vi "Proc_DCS.vi"(11 "error in (no error)":errorcluster, 12 "log file":path=path "/home/ArcVIEW/Logs/MOD_Logic_DCS.log", 13 "Database RefNum out":T1) -> (15 "error out":errorcluster)   [LabVIEW 2016]
uses:
  DBSHAND/private/vis/DatabaseHand_RefNum.ctl
  Common/public/vis/CMN_FVAR_action.ctl
  DBSHAND/private/vis/DatabaseHand_Element_Get(bool).vi
panel:
  out "queue":T2
  out "occurrence":refnum<k4>
  in  "input ptrs":u64[](array[numeric])
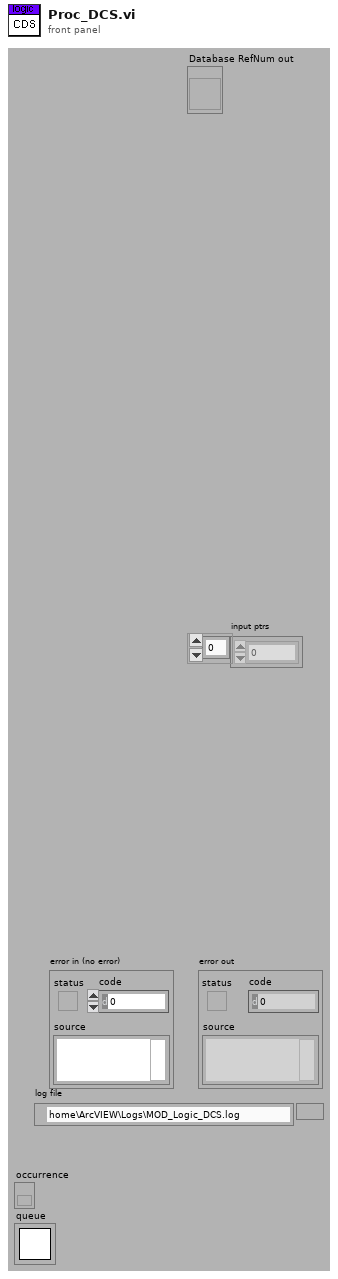
[diagram p1: front panel]
types:
  T1 = typedef "DatabaseHand_RefNum.ctl" = refnum<vi>
  T2 = typedef "Queue RefNum" = refnum<k1>
  T3 = typedef "CMN_FVAR_action.ctl" = enum16{"read", "write"}
  T4 = typedef "CMN_ContStatus.ctl" = cluster{"Response":string, "power":bool, "shutter":bool, "artifdata":bool, "idlemode":bool, "reset":bool, "gain":u8, "speed":u8, "resetPCI":bool, "autoshutter":bool, "TempSetPoint":i32, "multipleextensions":bool, "displayImage":bool, "coadding":bool, "images being coadded":i32, "Operation Mode":enum16{"normal", "coadd", "fawler"}, "frames to write":cluster{"subs":bool, "reset":bool, "exposed":bool}, "fawler samples":i32, "write auto":bool, "datatype":string, "frames to display":cluster{"subs":bool, "reset":bool, "exposed":bool}, "sur":i32, "autoclear":bool}
  T5 = typedef "CMN_Buffers.ctl" = cluster{"TotalPixels":u32, "Total image bytes":u32, "Total Phys Buffers":u32, "virtual buf pixels":u32, "virtual bytes size":u32, "Remaining piece":u32, "Transfer_Buf_size":u32}
  T6 = cluster{"subs":bool, "reset":bool, "exposed":bool}
  T7 = cluster{"name":string, "number":i32, "bpp":u8, "write ":bool, "imageToRead":u16, "rootName":string}
  T8 = cluster{"pointer":u64, "size":u64, "progress":u32, "status":string}
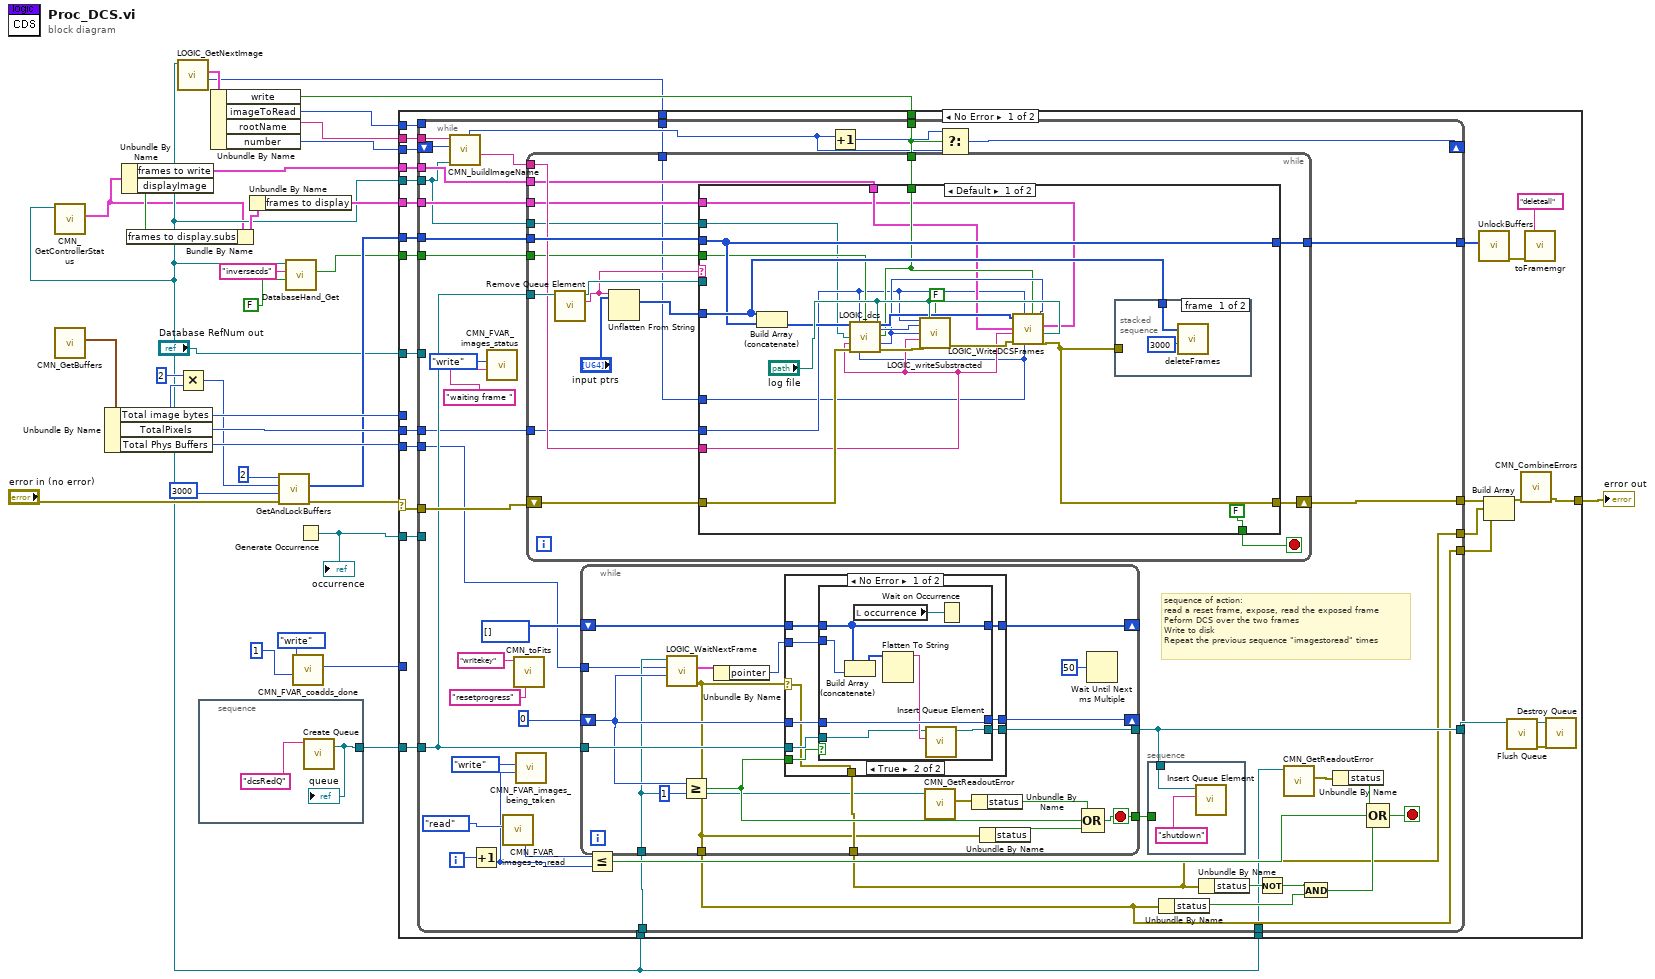
[diagram p0: block diagram]
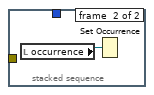
[diagram p2: hidden frame]
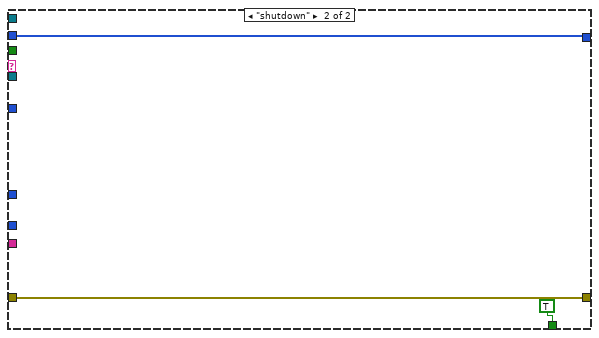
[diagram p3: hidden frame]
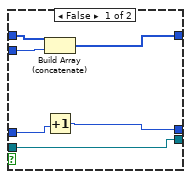
[diagram p4: hidden frame]
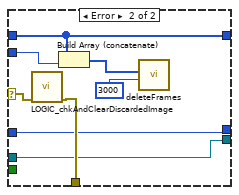
[diagram p5: hidden frame]
diagram:
  n1 = call "CMN_GetControllerStatus.vi"("DBS Ref"="Database RefNum out") -> ("ControllerStatus"=w3:T4)  [unwired: 10 out]
  n2 = call "CMN_GetBuffers.vi"() -> ("BuffersDimensions"=w5:T5)  [unwired: 2 in, 9 out]
  n3 = Unbundle By Name(w5) -> ("Total image bytes"=w28:u32, "TotalPixels"=w31:u32, "Total Phys Buffers"=w29:u32)
  n4 = Unbundle By Name(w3) -> ("frames to write"=w32:T6, "displayImage"=w14:bool)
  n5 = Bundle By Name(cluster=w3, "frames to display.subs"=w14) -> (w13:T4)
  n6 = call "LOGIC_GetNextImage.vi"("DBS Ref"="Database RefNum out") -> ("raw bpp"=w2:i32, "next image info"=w6:T7)  [unwired: 9 out]
  n7 = Multiply(x=u32 2, y=w28) -> (x*y=w24:u32)
  n8 = stacked-sequence {
    tunnel: [w33] -> w19
    frame #0 {
      n9 = call <vilib>:"Create Queue.vi"("name (unnamed)"="dcsRedQ") -> ("queue out"=w33:T2)  [unwired: 3 in, 3 out]
      "queue" <- w33
    }
  }
  n10 = Unbundle By Name(w6) -> ("write"=w17:bool, "imageToRead"=w18:u16, "rootName"=w16:string, "number"=w15:i32)
  n11 = Unbundle By Name(w13) -> ("frames to display"=w12:T6)
  n12 = call "GetAndLockBuffers.vi"("error in"="error in (no error)", "ms timeout (-1)"=3000, "size"=w24, "amount of buffers"=u16 2) -> ("error out"=w20:errorcluster, "ptrs"=w22:u64[])  [unwired: 1 in, 5 out]
  n13 = call-poly "DatabaseHand_Get.vi"("default value"=FALSE, "name"="inversecds", "Database RefNum in"="Database RefNum out") -> ("value"=w9:bool)  [unwired: 2 in, 6 out]
  n14 = call "CMN_FVAR_coadds_done.vi"("value in"=u16 1 ("images coadded"), "action"=CMN_FVAR_action."write") -> ("value out"=w1:i32)  [unwired: 8 out]
  n15 = Generate Occurrence() -> (w26:refnum<k4>)
  "occurrence" <- w26
  n16 = case shown="No Error" w20 {
    selector: w20 -> [w63 w205]
    tunnel: w32 -> [w58 _]
    tunnel: w31 -> [w36 _]
    tunnel: [w47 w205] -> w30
    tunnel: w29 -> [w53 _]
    tunnel: w26 -> [w59 _]
    tunnel: w22 -> [w62 _]
    tunnel: w19 -> [w60 _]
    tunnel: w28 -> [_ _]
    tunnel: w18 -> [w57 _]
    tunnel: w17 -> [w46 _]
    tunnel: "Database RefNum out" -> [w44 _]
    tunnel: "Database RefNum out" -> [w43 _]
    tunnel: "Database RefNum out" -> [w42 _]
    tunnel: w16 -> [w41 _]
    tunnel: w15 -> [w40 _]
    tunnel: w12 -> [w39 _]
    tunnel: w9 -> [w38 _]
    tunnel: "Database RefNum out" -> [w37 _]
    tunnel: w2 -> [w35 _]
    tunnel: w1 -> [_ _]
    frame No Error {
      n17 = while {
        tunnel: [w88] -> w45
        tunnel: w46 -> [w87]
        tunnel: [w91] -> w49
        tunnel: w53 -> [w65]
        tunnel: w57 -> [_]
        tunnel: w58 -> [w75]
        tunnel: w59 -> [_]
        tunnel: [w95] -> w56
        tunnel: w60 -> [w96]
        shift-left: w40 -> [w78]
        shift-right: [w85] -> _
        tunnel: w62 -> [w98]
        tunnel: [w99] -> w61
        tunnel: [w106] -> w50
        tunnel: w63 -> [w107]
        tunnel: w44 -> [w80]
        tunnel: w43 -> [w81]
        tunnel: w42 -> [w64]
        tunnel: w41 -> [w79]
        tunnel: w39 -> [w76]
        tunnel: w38 -> [w74]
        tunnel: w37 -> [_]
        tunnel: w36 -> [w67]
        tunnel: w35 -> [w66]
        i -> [w103]
        stop <- w100 stop-if-true
        # "sequence of action:\nread a reset frame, expose, read the exposed frame\nPeform DCS over the two frames\nWrite to disk\nRepeat the previous sequence \"imagestoread\" times"
        n18 = call "CMN_buildImageName.vi"("Database RefNum out"=w64, "imageNumber"=w78, "root name"=w79) -> ("image"=w97:string, "number"=w77:i32)  [unwired: 1 in, 4 out]
        n19 = Increment(x=w103) -> (x+1=w70:i32)
        n20 = call "CMN_FVAR_images_status.vi"("value in"="waiting frame " ("image status"), "action"=CMN_FVAR_action."write") -> ()  [unwired: 9 out]
        n21 = call "CMN_FVAR_images_to_read.vi"("action"=CMN_FVAR_action."read") -> ("value out"=w73:i32)  [unwired: 1 in, 8 out]
        n22 = call "CMN_toFits.vi"("key"="resetprogress", "command"="writekey") -> ()  [unwired: 6 in, 4 out]
        n23 = call "CMN_FVAR_images_being_taken.vi"("value in"=w70, "action"=CMN_FVAR_action."write") -> ()  [unwired: 9 out]
        n24 = while {
          tunnel: w87 -> [w115]
          tunnel: w97 -> [w114]
          tunnel: w98 -> [w118]
          tunnel: [w119] -> w99
          tunnel: w96 -> [w122]
          shift-left: w107 -> [w125]
          shift-right: [w124] -> w106
          tunnel: w76 -> [w112]
          tunnel: w75 -> [w113]
          tunnel: w74 -> [w111]
          tunnel: w67 -> [w110]
          tunnel: w66 -> [w109]
          tunnel: w64 -> [w108]
          stop <- w123 stop-if-true
          n25 = call <vilib>:"Remove Queue Element.vi"("queue"=w122) -> ("queue element"=w116:string, "queue out"=w117:T2)  [unwired: 2 in, 5 out]
          n26 = Unflatten From String(type="input ptrs", binary string=w116) -> (value=w120:u64[])  [unwired: 1 in, 4 out]
          n27 = case shown="Default" w116 {
            tunnel: w125 -> [w146 w152]
            tunnel: [w140 w152] -> w124
            tunnel: [FALSE TRUE] -> w123
            tunnel: w120 -> [w145 _]
            tunnel: [w144 w151] -> w119
            tunnel: w118 -> [w144 w151]
            tunnel: w117 -> [_ _]
            tunnel: w115 -> [w135 _]
            tunnel: w114 -> [w129 _]
            tunnel: w113 -> [w133 _]
            tunnel: w112 -> [w132 _]
            tunnel: w111 -> [w130 _]
            tunnel: w110 -> [w128 _]
            tunnel: w109 -> [w127 _]
            tunnel: w108 -> [w126 _]
            frame Default {
              n28 = Build Array (concatenate)(w145, w144) -> (w131:u64[])
              n29 = call "LOGIC_dcs.vi"("image ptrs (reset - expo - subs)"=w131, "TotalPixels"=w128, "inverse"=w130, "write to disk"=w135, "Database RefNum out 2"=w126, "Log File"="log file", "name"=w129, "error in (no error)"=w146, "reset and expo bpp"=w127) -> ("image ptrs (reset - expo - subs) out"=w141:u64[], "bpp"=w138:i16, "unsc buffer"=w137:u64, "error out"=w139:errorcluster)  [unwired: 3 out]
              n30 = call "LOGIC_writeSubstracted.vi"("total pixels"=w128, "log file"="log file", "write"=FALSE, "bpp"=w138, "subs buf"=w137, "name"=w129, "error in (no error)"=w139) -> ("error out"=w136:errorcluster)  [unwired: 8 out]
              n31 = call "LOGIC_WriteDCSFrames.vi"("log file"="log file", "frames to display"=w132, "unscramble ptr"=w137, "write to disk"=w135, "reset and expo bpp"=w127, "TotalPixels"=w128, "error in (no error)"=w136, "image name"=w129, "frames to write"=w133, "image ptrs (reset - expo)"=w141) -> ("error out"=w140:errorcluster)
              n32 = stacked-sequence {
                tunnel: w145 -> [w147 _]
                tunnel: w140 -> [_ _]
                frame #0 {
                  n33 = call "deleteFrames.vi"("ms timeout (-1)"=3000, "ptrs"=w147) -> ()  [unwired: 1 in, 9 out]
                }
                frame #1 {
                  n34 = local read "occurrence"() -> (w149:refnum<k4>)
                  n35 = Set Occurrence(w149) -> ()
                }
              }
            }
            frame "shutdown" {
            }
          }
        }
        n36 = while {
          tunnel: [w158] -> w88
          tunnel: [w164] -> w92
          tunnel: [w159] -> w91
          tunnel: [w166] -> w95
          tunnel: w96 -> [w167]
          shift-left: u64[] [] -> [w169]
          shift-right: [w168] -> _
          shift-left: 0 -> [w160]
          shift-right: [w171] -> _
          tunnel: w80 -> [w154]
          tunnel: w65 -> [w153]
          stop <- w164 stop-if-true
          n37 = call "LOGIC_WaitNextFrame.vi"("index"=w160, "total buffers"=w153, "Database RefNum in"=w154) -> ("error out"=w158:errorcluster, "frame ready"=w162:T8)  [unwired: 1 in, 6 out]
          n38 = Greater Or Equal?(x=w160, y=1) -> (x >= y?=w165:bool)
          n39 = Unbundle By Name(w162) -> ("pointer"=w161:u64)
          n40 = case shown="No Error" w158 {
            selector: w158 -> [w172 w202]
            tunnel: [w180 w200] -> w171
            tunnel: w169 -> [w179 w197]
            tunnel: [w178 w197] -> w168
            tunnel: w167 -> [w177 w199]
            tunnel: [w176 w199] -> w166
            tunnel: w165 -> [w175 _]
            tunnel: w161 -> [w174 w196]
            tunnel: w160 -> [w173 w200]
            tunnel: [w172 w201] -> w159
            frame No Error {
              n41 = case shown="True" w175 {
                tunnel: w174 -> [w186 w188]
                tunnel: [w185 w194] -> w180
                tunnel: w173 -> [w184 w194]
                tunnel: w179 -> [w183 w189]
                tunnel: [w182 w189] -> w178
                tunnel: w177 -> [w181 w192]
                tunnel: [w181 w191] -> w176
                frame False {
                  n42 = Build Array (concatenate)(w183, w186) -> (w182:u64[])
                  n43 = Increment(x=w184) -> (x+1=w185:i32)
                }
                frame True {
                  n44 = Build Array (concatenate)(w189, w188) -> (w187:u64[])
                  n45 = local read "occurrence"() -> (w190:refnum<k4>)
                  n46 = Flatten To String(anything=w187) -> (data string=w193:string)  [unwired: 1 in, 4 out]
                  n47 = call <vilib>:"Insert Queue Element.vi"("queue element"=w193, "queue"=w192) -> ("queue out"=w191:T2)  [unwired: 3 in, 4 out]
                  n48 = Wait on Occurrence(2:w190) -> ()  [unwired: 3 out]
                }
              }
            }
            frame Error {
              n49 = call "LOGIC_chkAndClearDiscardedImage.vi"("error in"=w202) -> ("error out"=w201:errorcluster)  [unwired: 10 out]
              n50 = Build Array (concatenate)(w197, w196) -> (w195:u64[])
              n51 = call "deleteFrames.vi"("ms timeout (-1)"=3000, "ptrs"=w195) -> ()  [unwired: 1 in, 9 out]
            }
          }
          n52 = call "CMN_GetReadoutError.vi"("Database RefNum in"=w154) -> ("readout_error"=w156:errorcluster)  [unwired: 1 in, 9 out]
          n53 = Unbundle By Name(w156) -> ("status"=w155:bool)
          n54 = Unbundle By Name(w158) -> ("status"=w157:bool)
          n55 = Compound Arithmetic op=OR(w155, w165, w157) -> (w164:bool)
          n56 = Wait Until Next ms Multiple(millisecond multiple=u32 50) -> ()  [unwired: 1 out]
        }
        n57 = Less Or Equal?(x=w73, y=w70) -> (x <= y?=w101:bool)
        n58 = Increment(x=w77) -> (x+1=w86:i32)
        n59 = Select(t=w86, s=w87, f=w77) -> (s? t:f=w85:i32)
        n60 = stacked-sequence {
          tunnel: w95 -> [w204]
          tunnel: w92 -> [_]
          frame #0 {
            n61 = call <vilib>:"Insert Queue Element.vi"("queue element"="shutdown", "queue"=w204) -> ()  [unwired: 3 in, 5 out]
          }
        }
        n62 = Unbundle By Name(w88) -> ("status"=w89:bool)
        n63 = Unbundle By Name(w91) -> ("status"=w93:bool)
        n64 = Not(x=w93) -> (.not. x?=w90:bool)
        n65 = call "CMN_GetReadoutError.vi"("Database RefNum in"=w81) -> ("readout_error"=w82:errorcluster)  [unwired: 1 in, 9 out]
        n66 = And(x=w90, y=w89) -> (x .and. y?=w94:bool)
        n67 = Unbundle By Name(w82) -> ("status"=w102:bool)
        n68 = Compound Arithmetic op=OR(w102, w101, w94) -> (w100:bool)
      }
      n69 = call "UnlockBuffers.vi"("ptrs in"=w61) -> ("error out"=w51:errorcluster)  [unwired: 2 in, 8 out]
      n70 = Build Array(w50, w49, w45) -> (w48:errorcluster[])
      n71 = call <vilib>:"Flush Queue.vi"("queue"=w56) -> ("error out"=w54:errorcluster, "queue out"=w55:T2)  [unwired: 1 in, 4 out]
      n72 = call "CMN_CombineErrors.vi"("Errors"=w48) -> ("error out"=w47:errorcluster)  [unwired: 10 out]
      n73 = call "toFramemgr.vi"("command"="deleteall", "error in"=w51) -> ()  [unwired: 7 in, 7 out]
      n74 = call <vilib>:"Destroy Queue.vi"("error in (no error)"=w54, "queue"=w55) -> ()  [unwired: 6 out]
    }
    frame Error {
    }
  }
  "error out" <- w30
